vi "flow rate timeseries data preprocessing (subVI).vi"() -> ()   [LabVIEW 2021]
uses:
  <vilib>/addons/Time Series Analysis/Series Preprocess.llb/TSA Vector Resampling (Unequal).vi
  <vilib>/addons/_Advanced Signal Processing/NI_AdvSigProcTSA.lvlib
panel:
  out "waveform []":waveform(dbl)[](array[waveform])
  in  "xy data []":cluster{"x":dbl[], "y":dbl[]}[](array[cluster])
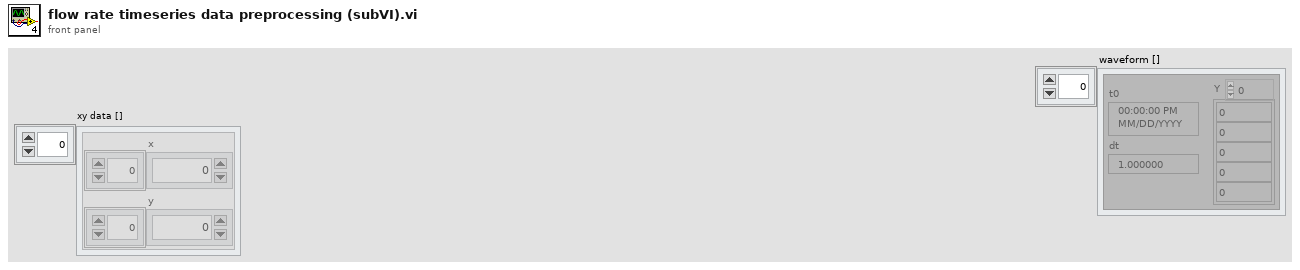
[diagram p1: front panel]
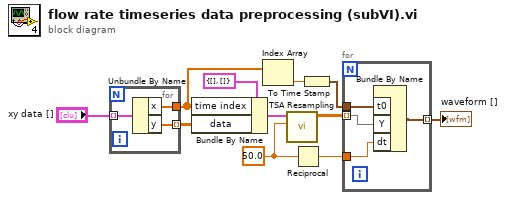
[diagram p0: block diagram]
diagram:
  w8 = 50.0 ("new sampling rate")
  n1 = for {
    tunnel: [w14] -> w2
    tunnel: [w13] -> w3 mode=indexing
    tunnel: "xy data []" -> [w12] mode=indexing
    n2 = Unbundle By Name(w12) -> ("x"=w14:dbl[], "y"=w13:dbl[])
  }
  n3 = Bundle By Name(cluster=cluster{"time index":dbl[], "data":dbl[][]} {"time index"=[], "data"=[]} ("Xt"), "time index"=w2, "data"=w3) -> (w10:cluster{"time index":dbl[], "data":dbl[][]})
  n4 = Index Array(array=w2) -> (element=w1:dbl)  [unwired: 1 in]
  n5 = call-poly <vilib>:"TSA Resampling.vi"("new sampling rate"=w8, "Xt"=w10) -> ("Xt resampled"=w9:dbl[][])  [unwired: 8 in, 1 out]
  n6 = Reciprocal(x=w8) -> (1/x=w7:dbl)
  n7 = To Time Stamp(1:w1) -> (0:w6:timestamp)
  n8 = for {
    tunnel: w9 -> [w18] mode=indexing
    tunnel: w7 -> [w17]
    tunnel: w6 -> [w16]
    tunnel: [w15] -> w4 mode=indexing
    n9 = Bundle By Name("t0"=w16, "Y"=w18, "dt"=w17) -> (w15:waveform(dbl))  [unwired: 1 in]
  }
  "waveform []" <- w4
